vi "Util_Progress Progress Popup with Status.vi"(10 "Message":string) -> ()   [LabVIEW 2013]
uses:
  App Images/TypeDefs/rad_Deployment Notifiers.ctl
  App Images/TypeDefs/rad_Deployment Status Data Type.ctl
  App Images/TypeDefs/rad_Deployment Progress Data Type.ctl
  FP Control/FP Control Functions.ctl
panel:
  in  "Deployment Notifiers":T1
  in  "Stop":bool
  out "Progress String":string="Transferring - This operation may take several minutes."
  out "Message out":string
  out "Progress":i32(slide) scale=0.0..100.0
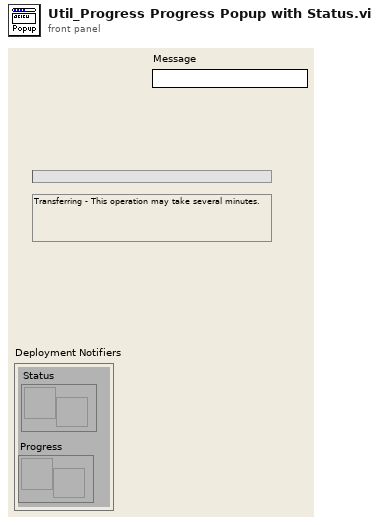
[diagram p1: front panel]
types:
  T1 = typedef "rad_Deployment Notifiers.ctl" = cluster{"Status":refnum<notifier>, "Progress":refnum<notifier>}
  T2 = typedef "FP Control Functions.ctl" = enum16{"Open", "Close", "Bring To Front", "Center"}
  T3 = typedef "rad_Deployment Progress Data Type.ctl" = i8
  T4 = typedef "rad_Deployment Status Data Type.ctl" = string
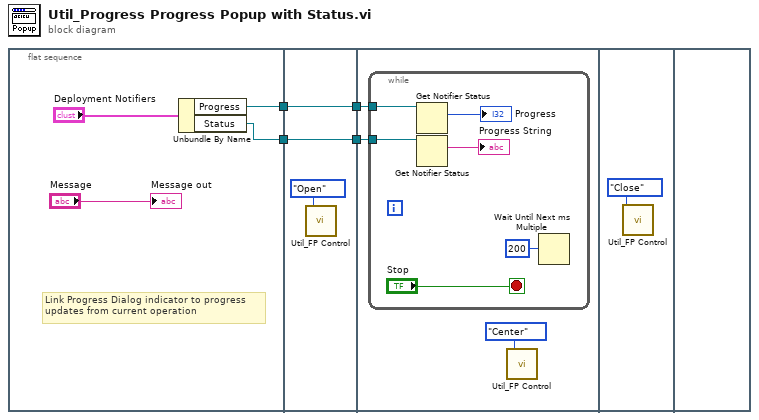
[diagram p0: block diagram]
diagram:
  n1 = flat-sequence {
    tunnel: [w6] -> w3
    tunnel: [w5] -> w1
    tunnel: [w10] -> w4
    tunnel: w3 -> [w10]
    tunnel: [w9] -> w2
    tunnel: w1 -> [w9]
    tunnel: w4 -> [w13]
    tunnel: w2 -> [w12]
    frame #0 {
      # "Link Progress Dialog indicator to progress\nupdates from current operation"
      n2 = Unbundle By Name("Deployment Notifiers") -> ("Progress"=w6:refnum<notifier>, "Status"=w5:refnum<notifier>)
      "Message out" <- "Message"
    }
    frame #1 {
      n3 = call "Util_FP Control.vi"("Function"=FP_Control_Functions."Open") -> ()  [unwired: 1 in, 10 out]
    }
    frame #2 {
      n4 = while {
        tunnel: w13 -> [w16]
        tunnel: w12 -> [w15]
        stop <- "Stop" stop-if-true
        n5 = Get Notifier Status(notifier=w16) -> (current notification=→"Progress":T3)  [unwired: 1 in, 4 out]
        n6 = Get Notifier Status(notifier=w15) -> (current notification=→"Progress String":T4)  [unwired: 1 in, 4 out]
        n7 = Wait Until Next ms Multiple(millisecond multiple=u32 200) -> ()  [unwired: 1 out]
      }
      n8 = call "Util_FP Control.vi"("Function"=FP_Control_Functions."Center") -> ()  [unwired: 1 in, 10 out]
    }
    frame #3 {
      n9 = call "Util_FP Control.vi"("Function"=FP_Control_Functions."Close") -> ()  [unwired: 1 in, 10 out]
    }
    frame #4 {
    }
  }
